vi "Apply on Cell.vi"(8 "error in":errorcluster, 10 "Cell":refnum<class "Cell.lvclass">, 11 "Cell View in":refnum<class "Cell View.lvclass">) -> (0 "error out":errorcluster, 3 "Cell View out":refnum<class "Cell View.lvclass">)   [LabVIEW 2024, in "SourceGrid.lvlib" / "Cell View.lvclass"]
doc: "Prepare and Set View to Cell"
uses:
  Cell View.lvclass
  Cell View.lvclass/Cell View.ctl
  Cells/Cell/Cell.lvclass
  D:/git/Sourcegrid-LabVIEW/dll/SourceGrid.dll
  dll/SourceGrid.dll
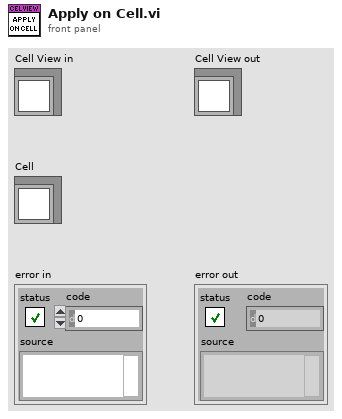
[diagram p1: front panel]
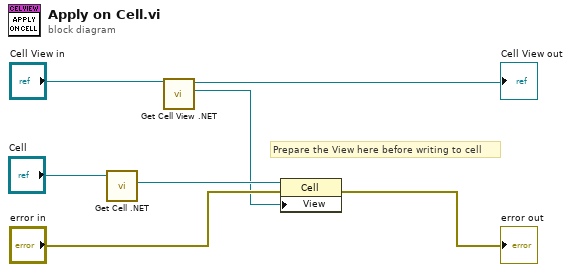
[diagram p0: block diagram]
diagram:
  # "Prepare the View here before writing to cell"
  n1 = call "Get Cell .NET.vi"("Cell in"="Cell") -> ("Cell .NET"=w5:refnum<k24>)  [unwired: 9 in, 1 out]
  n2 = call "Get Cell View .NET.vi"("Cell View in"="Cell View in") -> ("Cell View .NET"=w2:refnum<k24>, "Cell View out"=→"Cell View out":refnum<class "Cell View.lvclass">)  [unwired: 9 in]
  n3 = property class="Cell"(reference=w5, error in="error in", "View"=w2) -> (error out=→"error out":errorcluster)  [unwired: 1 out]
